vi "tvac_gui_v3.vi"() -> ()   [LabVIEW 2016]
uses:
  <vilib>/httpClient/LabVIEWHTTPClient.lvlib
  <vilib>/httpClient/ClientHandle.ctl
  <vilib>/httpClient/POSTBuffer.vi
  msg7171_linux.llb/send single message.vi
panel:
  out "Plot.Plot Color":u32
  in  "alarm":i32
  out "String 2":string
  in  "Tab Control":enum32{"Page 1", "Page 2"}(tab)
  in  "Zone 1":T1 {"Ring" items=["Average", "Maximum", "Minimum", ""]}
  out "Thermocouple":T2(array[cluster]) {"Numeric" format="%#.2g"}
  out "Waveform Chart":waveform(dbl)[](graph)
  in  "exit":bool
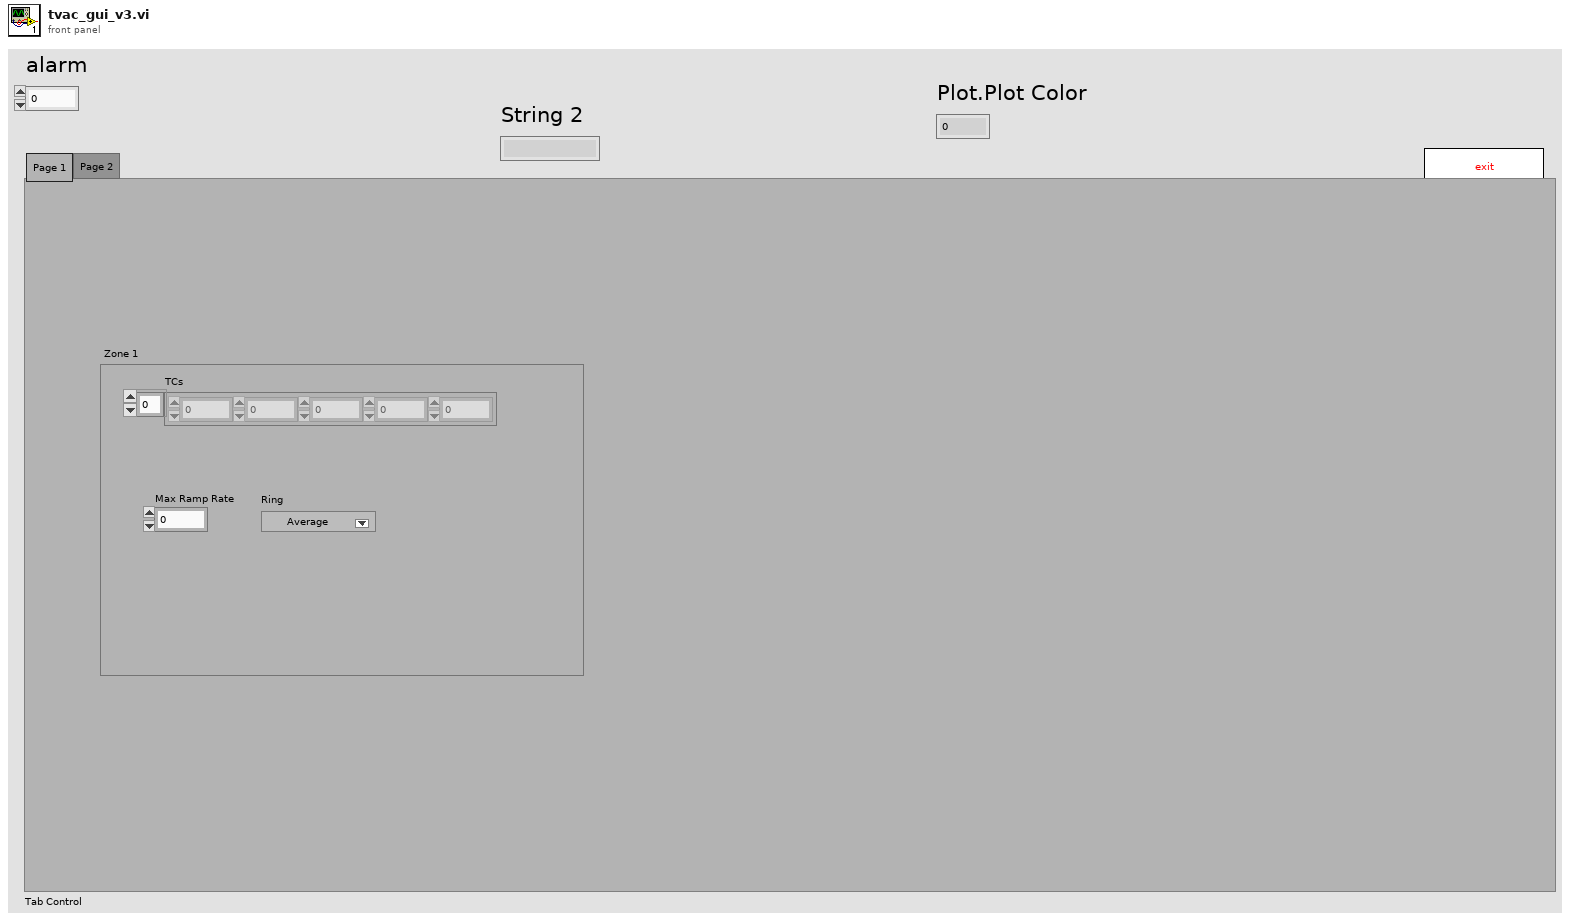
[diagram p1: front panel]
types:
  T1 = cluster{"Ring":u16, "Max Ramp Rate":dbl, "TCs":dbl[]}
  T2 = cluster{"Numeric":dbl, "Color Box":u32, "String":string, "PlotColor":u32}[][]
  T3 = typedef "LabVIEWHTTPClient.lvlib/ClientHandle.ctl" = refnum<k1>
  T4 = cluster{"go":bool, "Http session":T3, "URL prefex":string}
  T5 = typedef "LVPoint32TypeDef.ctl" = cluster{"Horizontal":i32, "Vertical":i32}
  T6 = typedef "LVPositionTypeDef.ctl" = cluster{"Left":i32, "Top":i32}
  T7 = cluster{"Numeric":dbl, "Color Box":u32, "String":string, "PlotColor":u32}
  T8 = cluster{"time":string, "tcs":cluster{"thermocouple":i32, "time":i32, "temp":i32, "working":i32, "alarm":i32}[]}
  T9 = cluster{"thermocouple":i32, "time":i32, "temp":i32, "working":i32, "alarm":i32}[]
  T10 = cluster{"thermocouple":i32, "time":i32, "temp":i32, "working":i32, "alarm":i32}
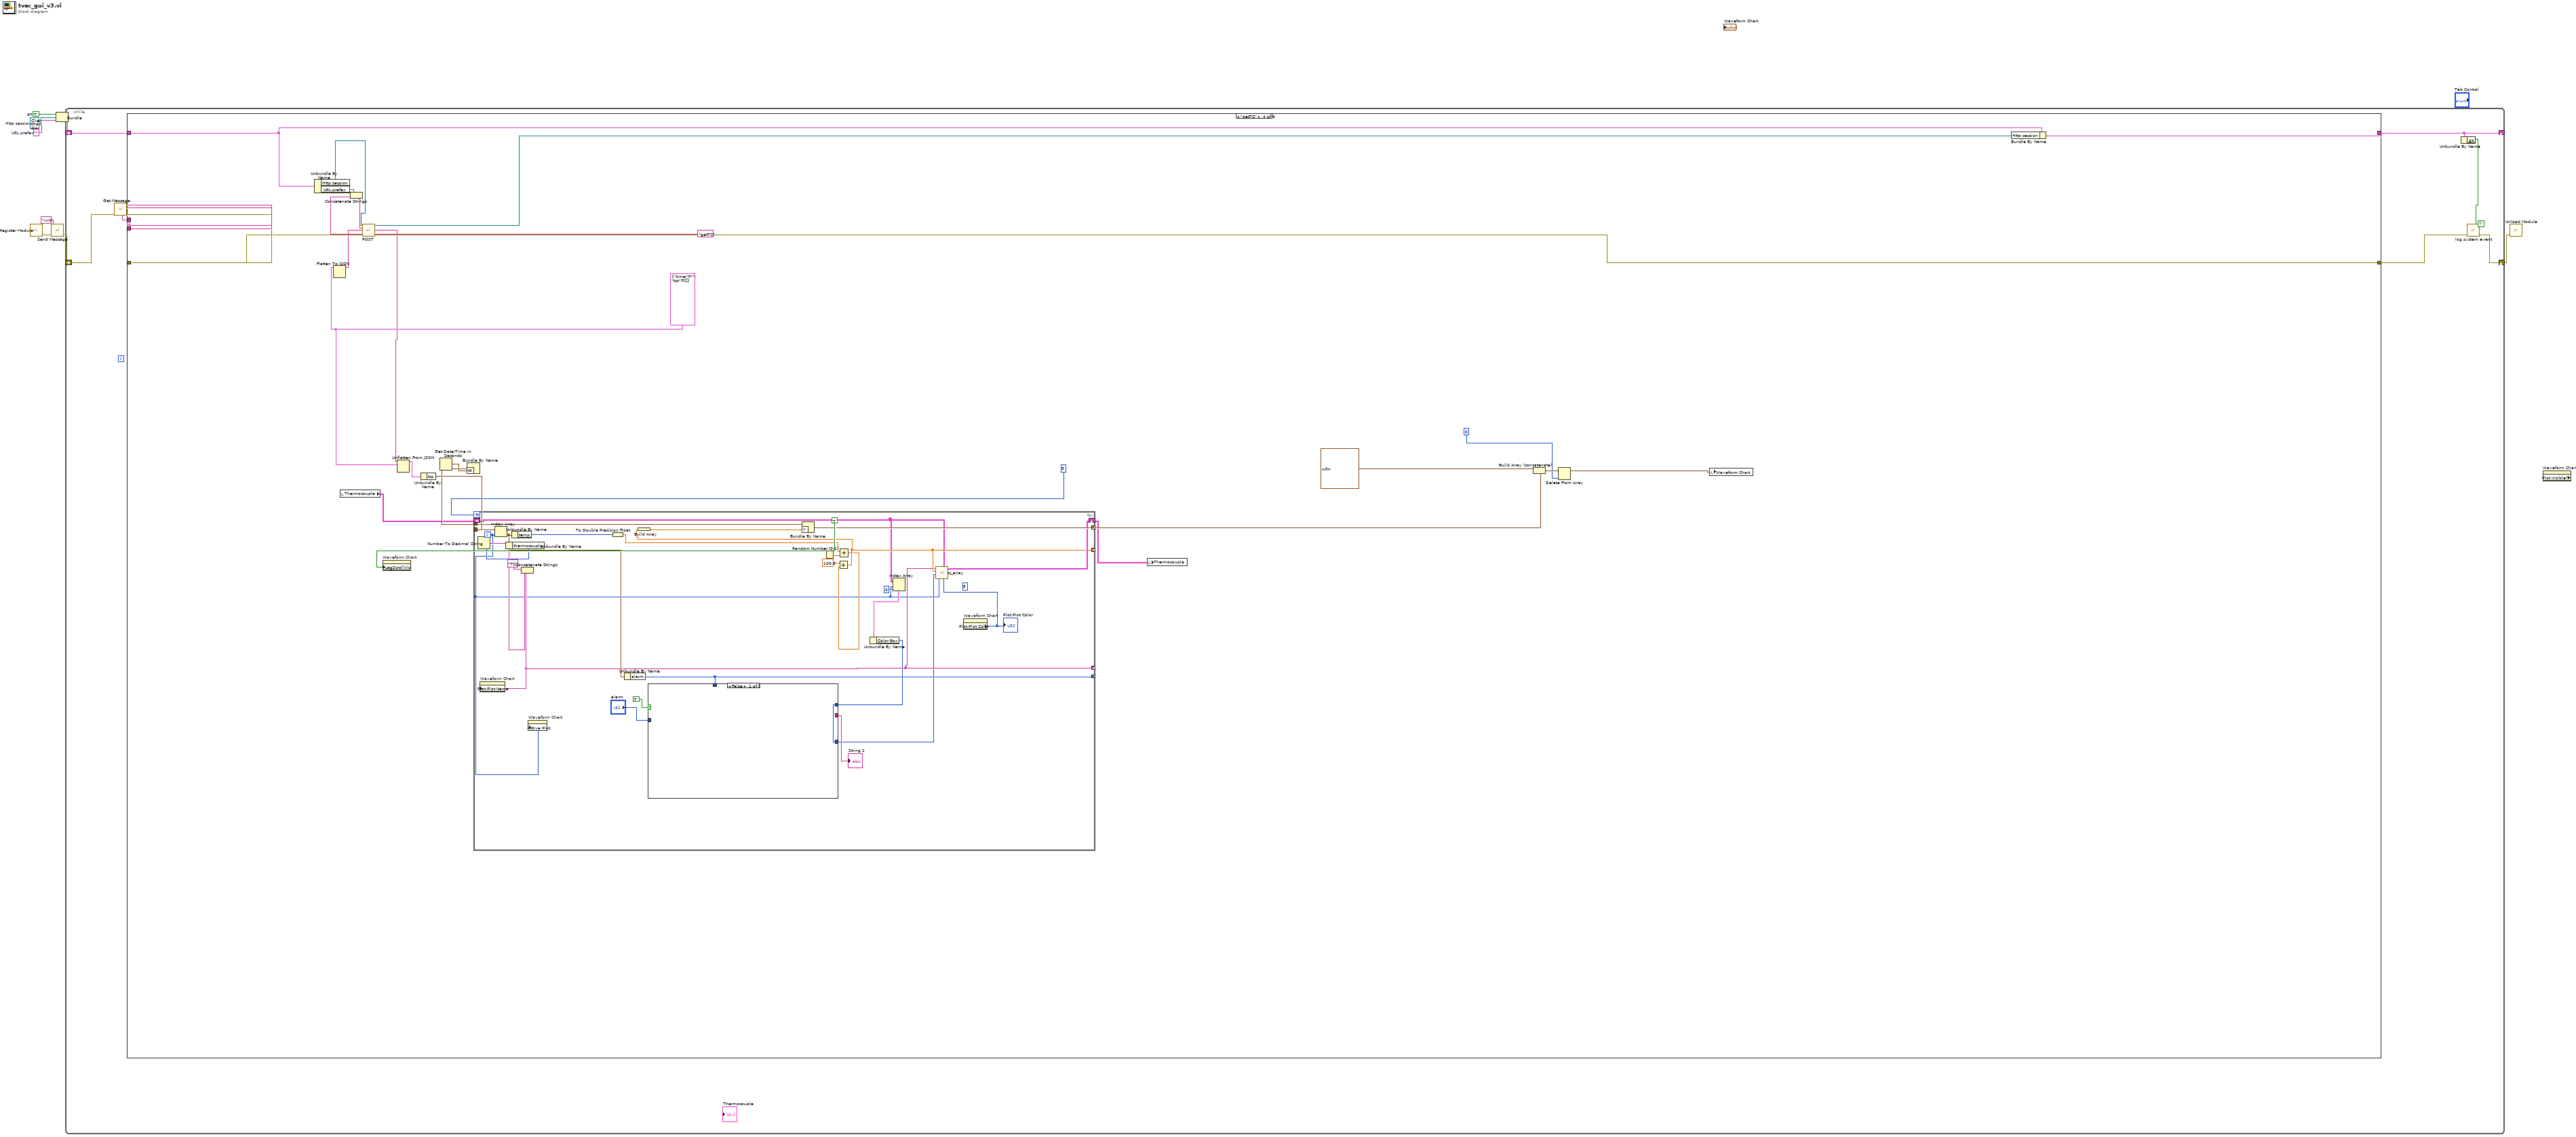
[diagram p0: block diagram]
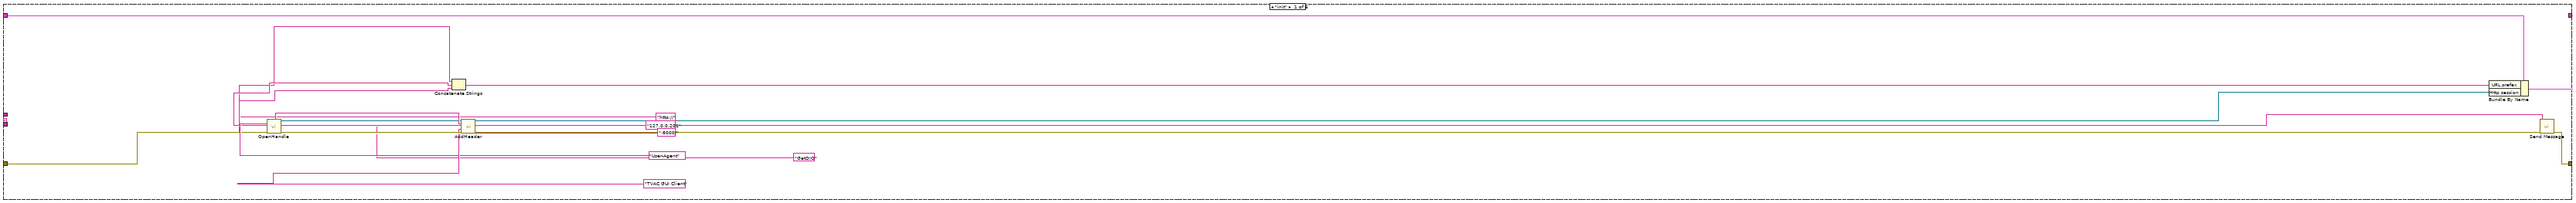
[diagram p2: hidden frame]
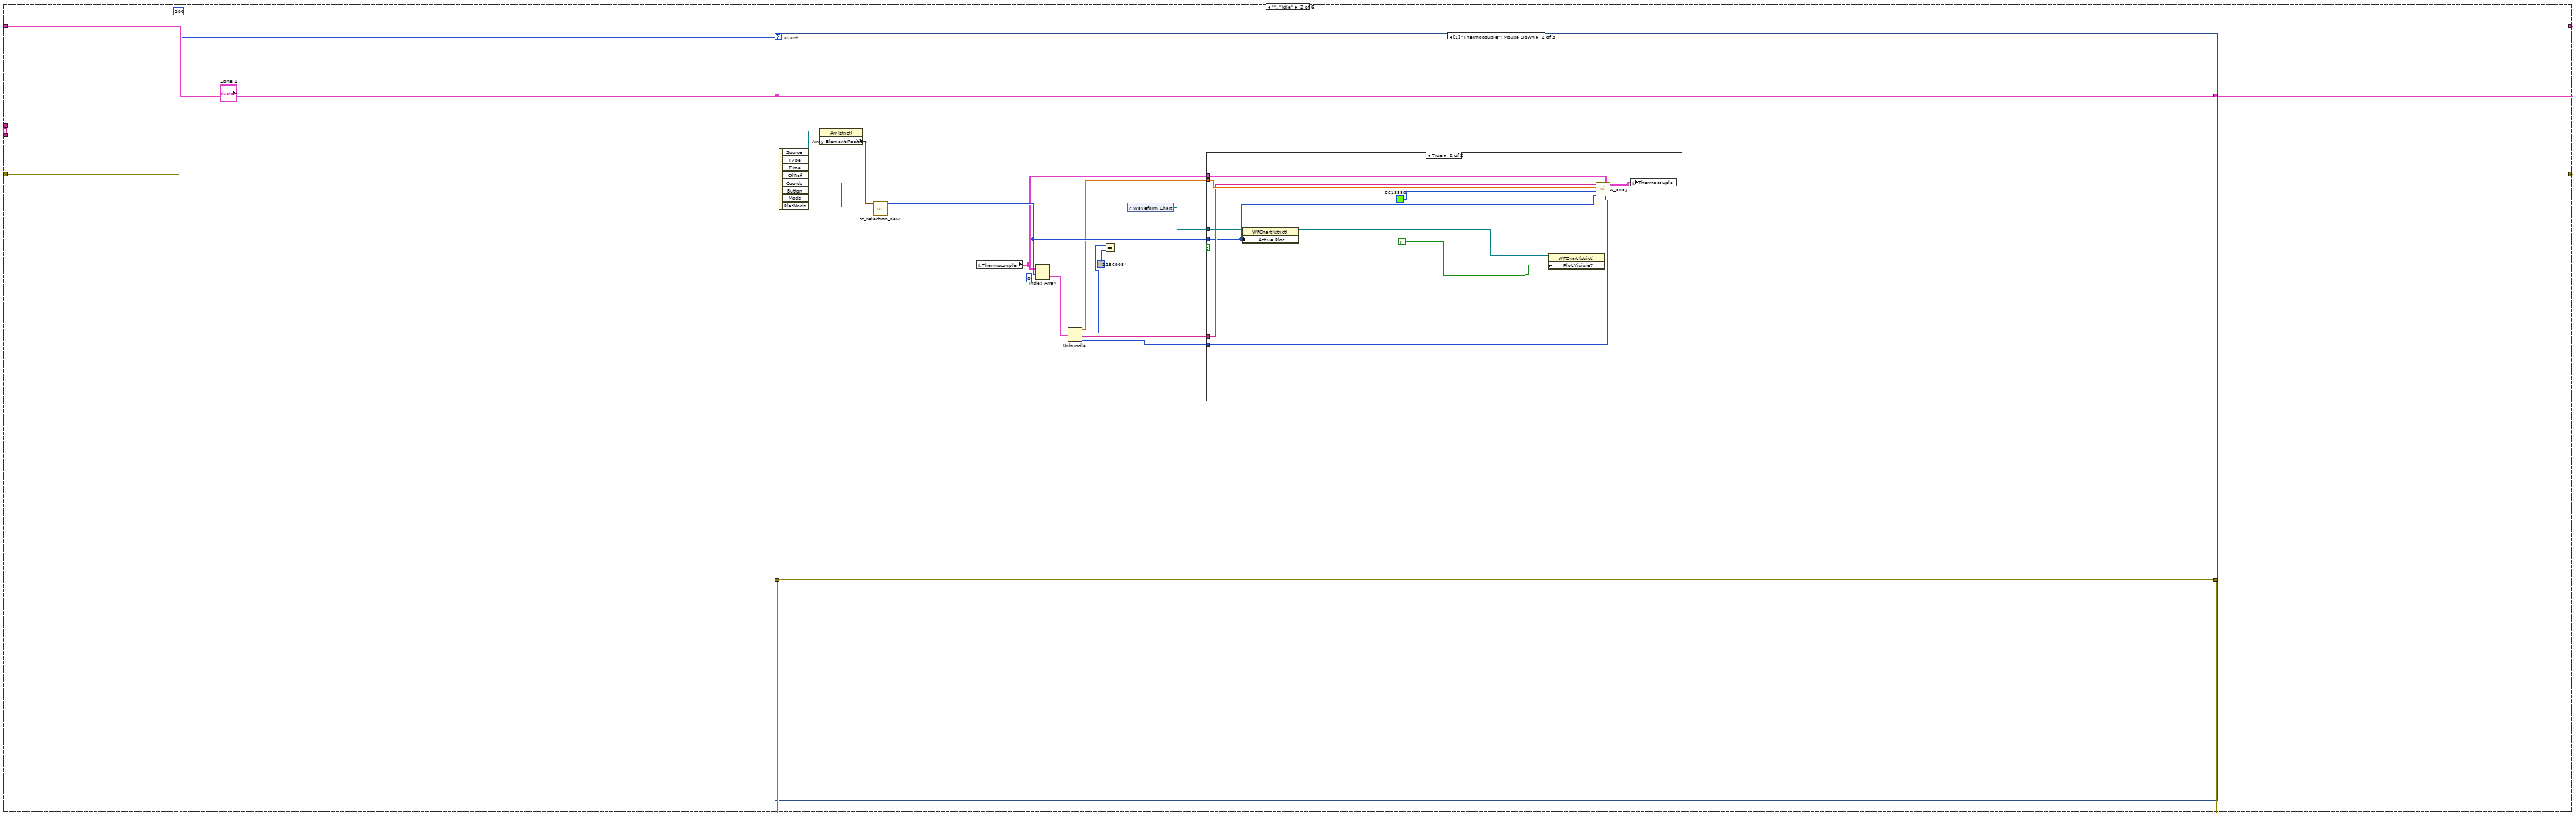
[diagram p3: hidden frame]
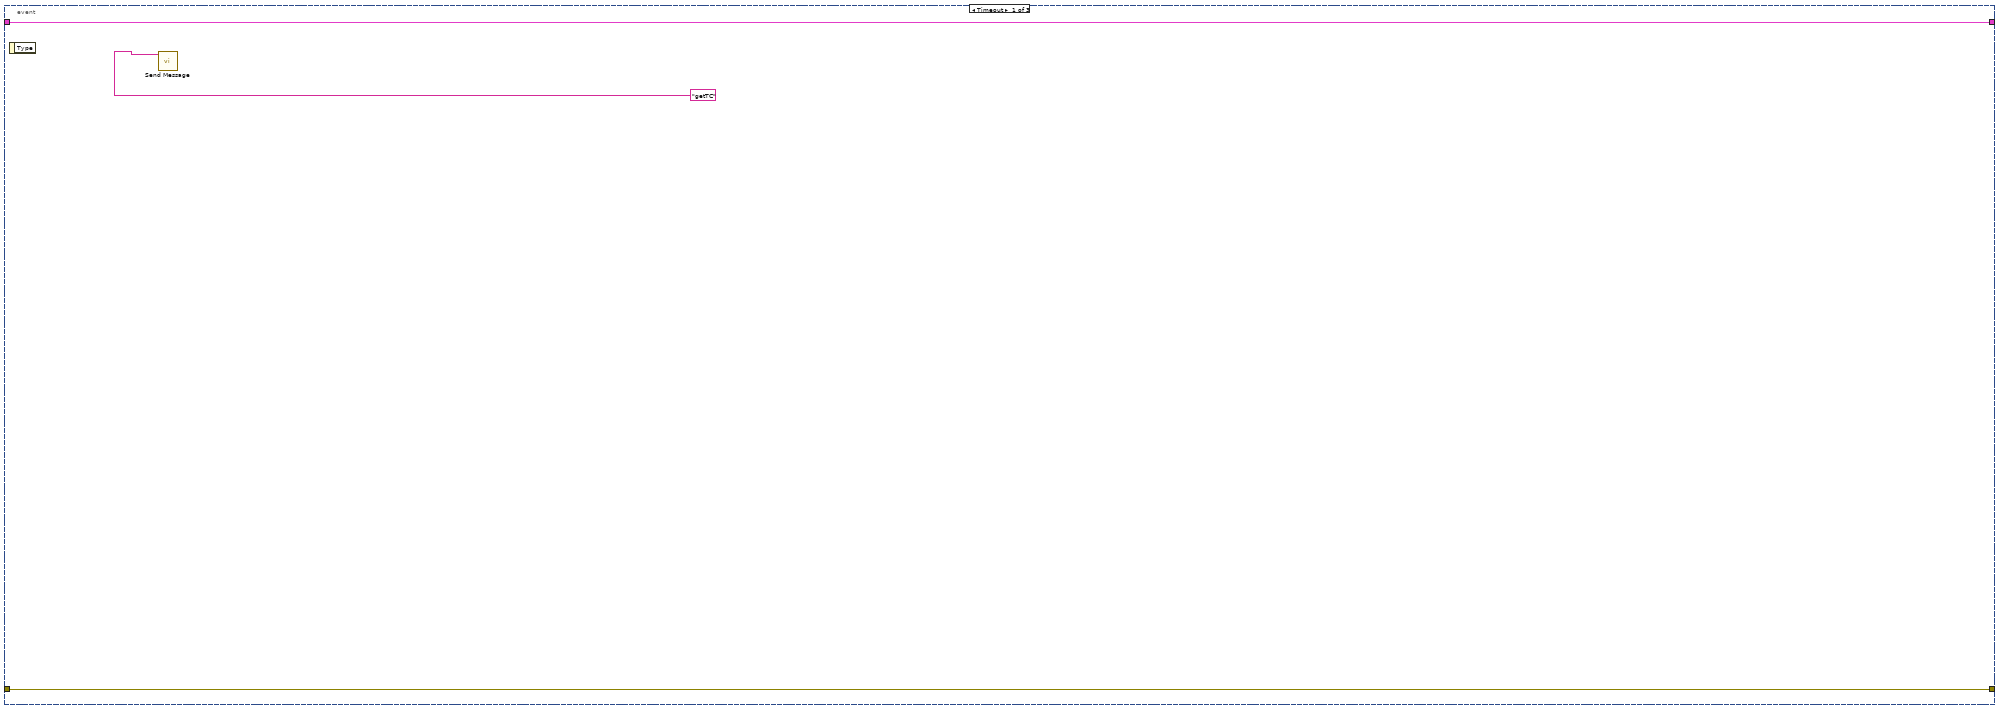
[diagram p4: hidden frame]
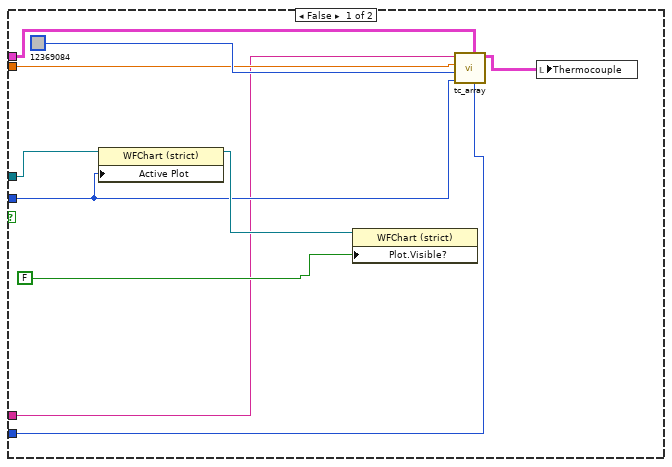
[diagram p5: hidden frame]
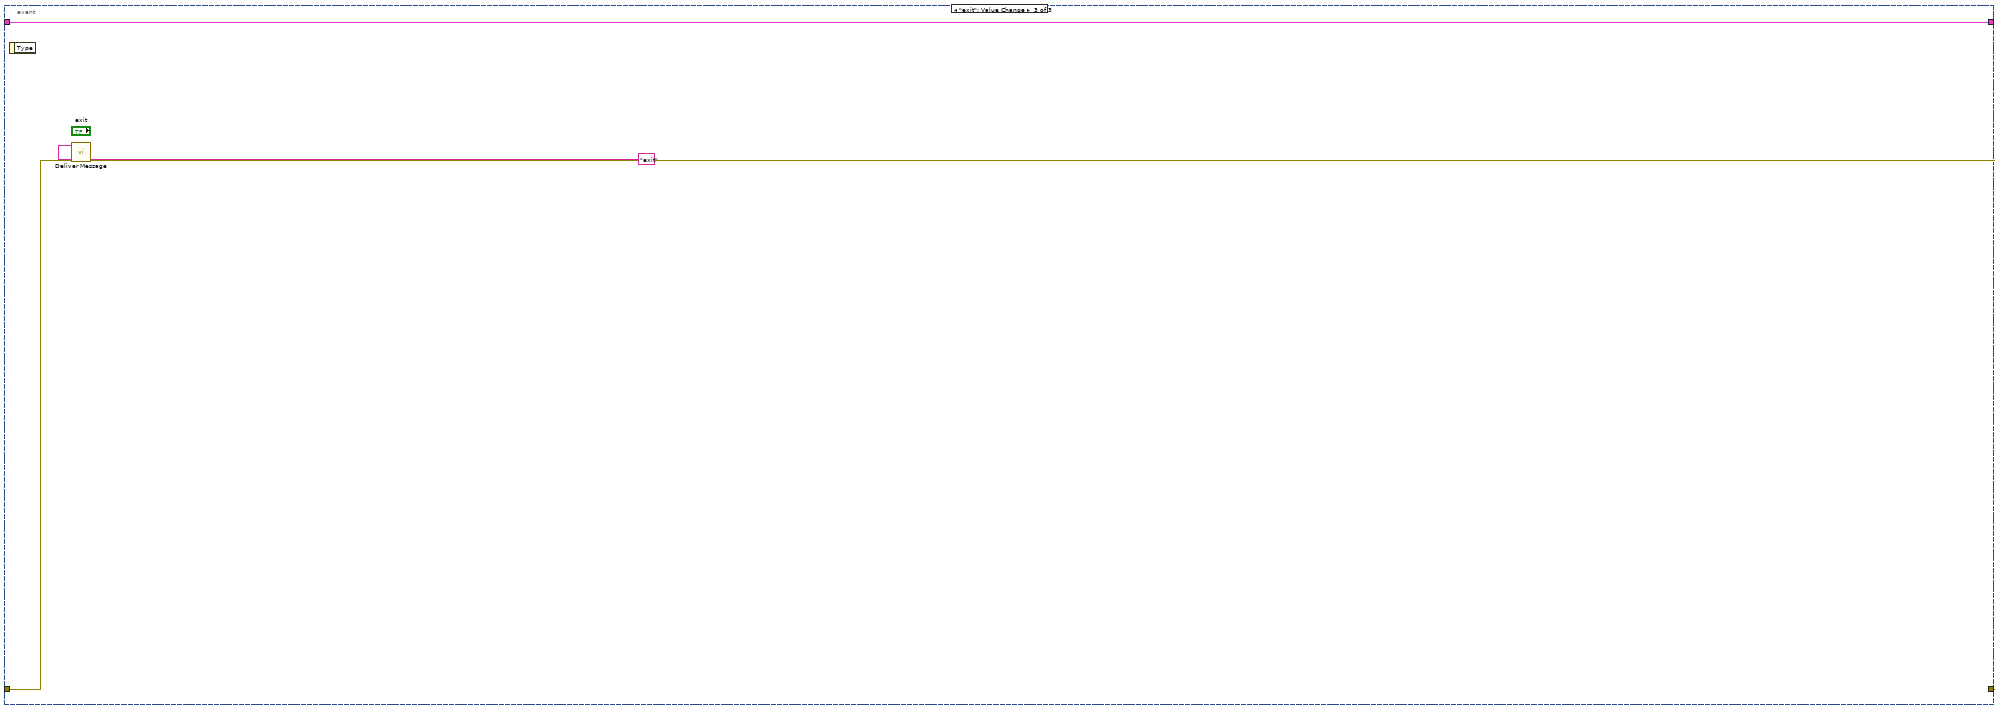
[diagram p6: hidden frame]
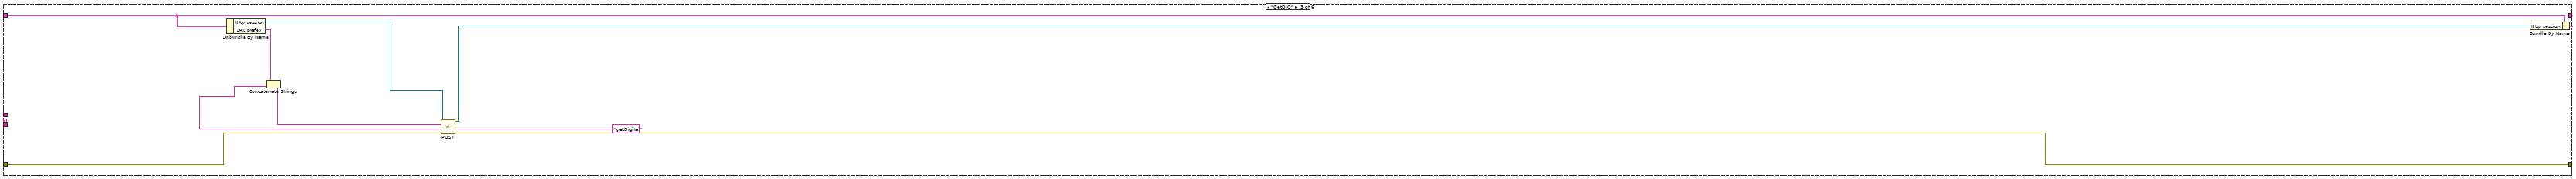
[diagram p7: hidden frame]
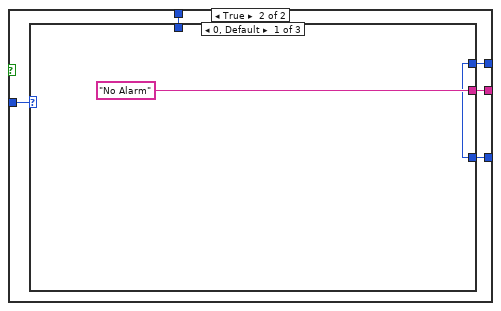
[diagram p8: hidden frame]
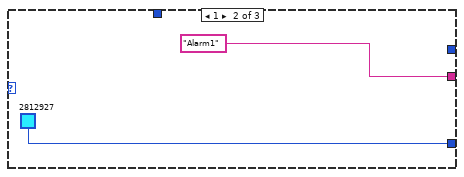
[diagram p9: hidden frame]
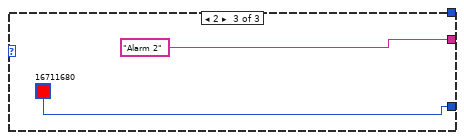
[diagram p10: hidden frame]
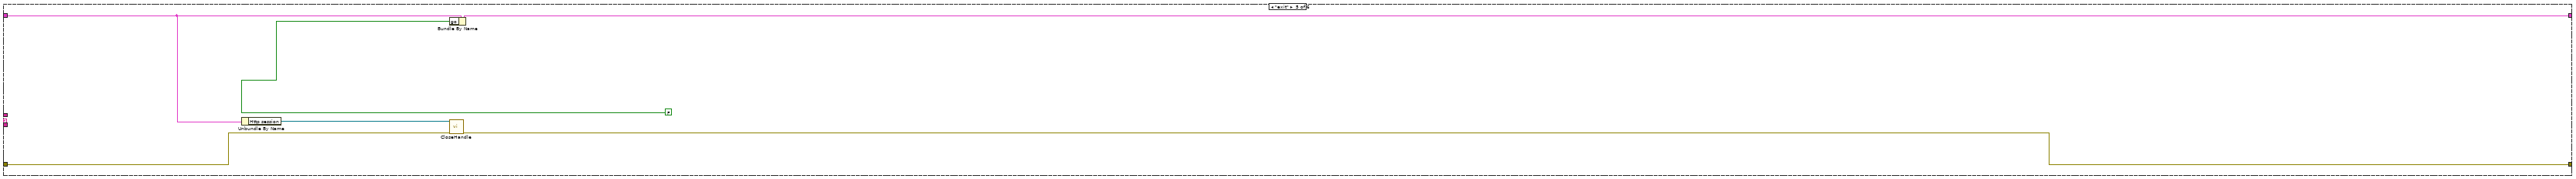
[diagram p11: hidden frame]
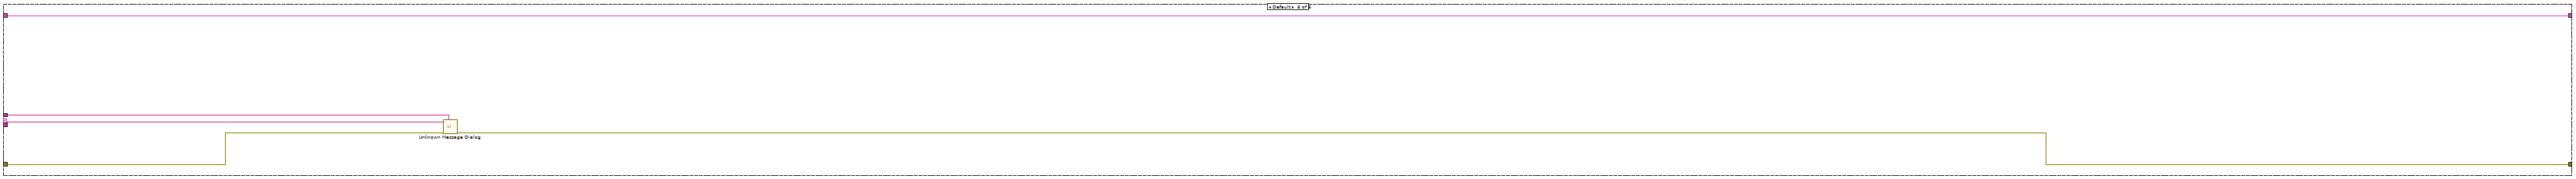
[diagram p12: hidden frame]
diagram:
  w4 = ""  # URL prefex
  w5 = T3 refnum  # Http session
  w6 = TRUE  # go
  n1 = call "Register Module.vi"() -> ("error out"=w2:errorcluster)  [unwired: 10 in, 1 out]
  n2 = call-poly "Send Message.vi"("error in (no error)"=w2, "event"="init") -> ("error out"=w1:errorcluster)  [unwired: 9 in]
  n3 = Bundle("go"=w6, "Http session"=w5, "URL prefex"=w4) -> (w8:T4)  [unwired: 1 in]
  n4 = while {
    shift-left: w8 -> [w15]
    shift-right: [w12] -> _
    shift-right: [w10] -> w7
    shift-left: w1 -> [w18]
    stop <- w11 continue-if-true
    n5 = call "Get Message.vi"("error in (no error)"=w18) -> ("error out"=w16:errorcluster, "event buffer"=w17:string, "event"=w14:string, "source"=w13:string)  [unwired: 7 in]
    n6 = case shown="\"getTC\"" w14 {
      selector: w14 -> [_ _ _ _ _ w163]
      tunnel: [w24 w35 w83 w113 w160 w165] -> w12
      tunnel: w15 -> [w33 w34 w82 w111 w155 w165]
      tunnel: w17 -> [_ _ _ _ _ _]
      tunnel: w16 -> [w28 w36 w85 w115 w158 w164]
      tunnel: w13 -> [_ _ _ _ _ w162]
      tunnel: [w20 w38 w84 w114 w157 w161] -> w9
      frame "init" {
        n7 = call <vilib>:"OpenHandle.vi"("error in (no error)"=w28) -> ("client handle out"=w29:T3, "error out"=w32:errorcluster)  [unwired: 13 in]
        n8 = Concatenate Strings("http://" ("url"), "127.0.0.201" ("Address"), ":8000/" ("url")) -> (w23:string)
        n9 = call <vilib>:"AddHeader.vi"("client handle"=w29, "header"="User-Agent", "value"="TVAC GUI Client", "error in (no error)"=w32) -> ("client handle out"=w22:T3, "error out"=w21:errorcluster)  [unwired: 10 in]
        n10 = Bundle By Name(cluster=w33, "URL prefex"=w23, "Http session"=w22) -> (w24:T4)
        n11 = call-poly "Send Message.vi"("error in (no error)"=w21, "event"="GetDIO") -> ("error out"=w20:errorcluster)  [unwired: 9 in]
      }
      frame "", "Idle" {
        n12 = event shown="[1] \"Thermocouple\": Mouse Down" {
          selector: _ -> [_ _ _]
          dyn-events: _ -> [_ _ _]
          timeout: 200 ("milliseconds to wait") -> [_ _ _]
          tunnel: w36 -> [w40 w57 w81]
          tunnel: [w40 w57 w80] -> w38
          tunnel: [w41 w56 w78] -> w35
          tunnel: w34 -> [w41 w56 w78]
          event Timeout {
            n13 = event-data() -> ()  [unwired: 1 in, 1 out]
            n14 = call-poly "Send Message.vi"("event"="getTC") -> ()  [unwired: 10 in, 1 out]
          }
          event "Thermocouple": Mouse Down {
            n15 = event-data() -> ("CtlRef"=w53:refnum<vi>, "Coords"=w54:T5)  [unwired: 1 in, 6 out]
            n16 = property class="Arr (strict)"(reference=w53) -> ("Array Element.Position"=w55:T6)  [unwired: 1 in, 2 out]
            n17 = call "tc_selection_new.vi"("Coords"=w54, "Position"=w55) -> ("Numeric"=w47:i32)  [unwired: 9 in]
            n18 = local read "Thermocouple"() -> (w45:T2)
            n19 = Index Array(array=w45, index (row)=w47, index (col)=0 ("disabled index (col)")) -> (element=w50:T7)
            n20 = Unbundle(w50) -> ("Numeric"=w44:dbl, "Color Box"=w49:u32, "String"=w43:string, "PlotColor"=w42:u32)
            n21 = Equal?(x=w49, y=u32 12369084) -> (x = y?=w48:bool)
            n22 = control-ref of="Waveform Chart"() -> (w46:refnum<vi>)
            n23 = case shown="True" w48 {
              tunnel: w47 -> [w64 w72]
              tunnel: w46 -> [w65 w75]
              tunnel: w45 -> [w58 w69]
              tunnel: w44 -> [w62 w74]
              tunnel: w43 -> [w61 w73]
              tunnel: w42 -> [w59 w70]
              frame False {
                n24 = property on="Property Node" class="WFChart (strict)"(reference=w65, "Active Plot"=w64) -> (reference out=w66:refnum<vi>)  [unwired: 1 in, 1 out]
                n25 = property class="WFChart (strict)"(reference=w66, "Plot.Visible?"=FALSE ("Plot.Visible")) -> ()  [unwired: 1 in, 2 out]
                n26 = call "tc_array.vi"("String"=w61, "Numeric"=w62, "Color Box"=u32 12369084, "index (row)"=w64, "output array 2"=w58, "PlotColor"=w59) -> ("output array"=w60:T2)  [unwired: 3 in]
                n27 = local write "Thermocouple"(w60) -> ()
              }
              frame True {
                n28 = property class="WFChart (strict)"(reference=w75, "Active Plot"=w72) -> (reference out=w76:refnum<vi>)  [unwired: 1 in, 1 out]
                n29 = property class="WFChart (strict)"(reference=w76, "Plot.Visible?"=TRUE ("Plot.Visible")) -> ()  [unwired: 1 in, 2 out]
                n30 = call "tc_array.vi"("String"=w73, "Numeric"=w74, "Color Box"=u32 6618880, "index (row)"=w72, "output array 2"=w69, "PlotColor"=w70) -> ("output array"=w68:T2)  [unwired: 3 in]
                n31 = local write "Thermocouple"(w68) -> ()
              }
            }
          }
          event "exit": Value Change {
            n32 = event-data() -> ()  [unwired: 1 in, 1 out]
            n33 = call "Deliver Message.vi"("error in (no error)"=w81, "event"="exit") -> ("error out"=w80:errorcluster)  [unwired: 9 in]
          }
        }
      }
      frame "GetDIO" {
        n34 = Unbundle By Name(w82) -> ("Http session"=w89:T3, "URL prefex"=w87:string)
        n35 = Concatenate Strings(w87, "getDigital" ("url")) -> (w88:string)
        n36 = call-poly <vilib>:"POST.vi"("client handle"=w89, "url"=w88, "error in (no error)"=w85) -> ("client handle out"=w90:T3, "error out"=w84:errorcluster)  [unwired: 9 in, 2 out]
        n37 = Bundle By Name(cluster=w82, "Http session"=w90) -> (w83:T4)
      }
      frame "getTC" {
        w104 = T8 {"time"="", "tcs"=[]}
        n38 = Unbundle By Name(w111) -> ("Http session"=w110:T3, "URL prefex"=w108:string)
        n39 = Flatten To JSON(anything=w104) -> (JSON string=w106:string)  [unwired: 2 in, 1 out]
        n40 = local read "Thermocouple"() -> (w93:T2)
        n41 = Concatenate Strings(w108, "getTC" ("url")) -> (w109:string)
        n42 = call-poly <vilib>:"POST.vi"("client handle"=w110, "url"=w109, "buffer"=w106, "error in (no error)"=w115) -> ("client handle out"=w112:T3, "body"=w105:string, "error out"=w114:errorcluster)  [unwired: 8 in, 1 out]
        n43 = property on="Waveform Chart" class="WFChart (strict)"("LegScrollVis"=TRUE ("Legend:Scrollbar Visible")) -> ()  [unwired: 2 in, 2 out]
        n44 = Unflatten From JSON(JSON string=w105, type and defaults=w104) -> (value=w103:T8)  [unwired: 5 in, 1 out]
        n45 = Unbundle By Name(w103) -> ("tcs"=w102:T9)
        n46 = Get Date/Time In Seconds() -> (seconds since 1Jan1904=w98:timestamp)
        n47 = Bundle By Name("t0"=w98) -> (w97:waveform(dbl))  [unwired: 1 in]
        n48 = for {
          N: 5 -> [_]
          tunnel: w102 -> [w142]
          tunnel: w97 -> [w140]
          tunnel: [w141] -> w96 mode=indexing
          tunnel: [w122] -> _ mode=indexing
          tunnel: [w121] -> _ mode=indexing
          tunnel: [w124] -> _ mode=indexing
          shift-right: [w123] -> w94
          shift-left: w93 -> [w120]
          i -> [w119]
          (unwired) 5
          n49 = Index Array(array=w142, index=w119) -> (element=w132:T10)
          n50 = Unbundle By Name(w132) -> ("thermocouple"=w138:i32)
          n51 = Number To Decimal String(number=w138) -> (decimal integer string=w139:string)  [unwired: 1 in]
          n52 = Unbundle By Name(w132) -> ("temp"=w136:i32)
          n53 = Concatenate Strings("TC " ("string"), w139) -> (w121:string)
          n54 = property on="Waveform Chart" class="WFChart (strict)"("Plot.Plot Name"=w121) -> ()  [unwired: 2 in, 2 out]
          n55 = property on="Waveform Chart" class="WFChart (strict)"("Active Plot"=w119) -> ()  [unwired: 2 in, 2 out]
          n56 = To Double Precision Float(number=w136) -> (double precision float=w133:dbl)
          n57 = Unbundle By Name(w132) -> ("alarm"=w124:i32)
          n58 = Random Number (0-1)() -> (number: 0 to 1=w134:dbl)
          n59 = Add(x=w133, y=w134) -> (x+y=w130:dbl)
          n60 = Add(x=100.0, y=w130) -> (x+y=w122:dbl)
          n61 = Build Array(w122) -> (w135:dbl[])
          n62 = Bundle By Name(cluster=w140, "Y"=w135) -> (w141:waveform(dbl))
          n63 = Index Array(array=w120, index (row)=w119, index (col)=0 ("disabled index (col)")) -> (element=w127:T7)
          n64 = Unbundle By Name(w127) -> ("Color Box"=w116:u32)
          n65 = case shown="False" TRUE {
            tunnel: [_ w148] -> w129
            tunnel: "alarm" -> [_ w147]
            tunnel: w124 -> [_ w146]
            tunnel: [w143 w145] -> w117
            tunnel: w116 -> [w143 w144]
            frame False {
            }
            frame True {
              n66 = case shown="0, Default" w147 {
                tunnel: ["No Alarm" "Alarm1" "Alarm 2"] -> w148
                tunnel: w146 -> [_ _ _]
                tunnel: [w149 u32 2812927 u32 16711680] -> w145
                tunnel: w144 -> [w149 _ _]
                frame 0, Default {
                }
                frame 1 {
                }
                frame 2 {
                }
              }
            }
          }
          "String 2" <- w129
          n67 = property on="Waveform Chart" class="WFChart (strict)"() -> ("Plot.Plot Color"=w118:u32)  [unwired: 2 in, 2 out]
          "Plot.Plot Color" <- w118
          n68 = call "tc_array.vi"("String"=w121, "Numeric"=w122, "Color Box"=w117, "index (row)"=w119, "output array 2"=w120, "PlotColor"=w118) -> ("output array"=w123:T2)  [unwired: 3 in]
        }
        n69 = local write "Thermocouple"(w94) -> ()
        n70 = Build Array (concatenate)(waveform(dbl) {"t0"=timestamp(0 s since 1904-01-01), "dt"=1.0, "Y"=[]} ("element"), w96) -> (w100:waveform(dbl)[])
        n71 = Delete From Array(array=w100, index=0) -> (array with subset deleted=w91:waveform(dbl)[])  [unwired: 1 in, 1 out]
        n72 = local write "Waveform Chart"(w91) -> ()
        n73 = Bundle By Name(cluster=w111, "Http session"=w112) -> (w113:T4)
      }
      frame "exit" {
        n74 = Unbundle By Name(w155) -> ("Http session"=w156:T3)
        n75 = Bundle By Name(cluster=w155, "go"=FALSE ("Bundle Element")) -> (w160:T4)
        n76 = call <vilib>:"CloseHandle.vi"("client handle"=w156, "error in (no error)"=w158) -> ("error out"=w157:errorcluster)  [unwired: 13 in]
      }
      frame Default {
        n77 = call "Unknown Message Dialog.vi"("source"=w162, "error in (no error)"=w164, "event name"=w163) -> ("error out"=w161:errorcluster)  [unwired: 8 in]
      }
    }
    n78 = Unbundle By Name(w12) -> ("go"=w11:bool)
    n79 = call "log system event.vi"("error in (no error)"=w9) -> ("error out"=w10:errorcluster)  [unwired: 9 in, 1 out]
  }
  n80 = call "Unload Module.vi"("error in (no error)"=w7) -> ()  [unwired: 10 in, 1 out]
  n81 = property on="Waveform Chart" class="WFChart (strict)" props=["Plot", "Visible?"]() -> ()  [unwired: 2 in, 3 out]
